vi "Edit Row.vi"(6 "Row Index":i32, 8 "error in (no error)":errorcluster, 9 "New Row Data (or multi rows)":string[][](array[string]), 11 "DataGrid.lvlib:DataTable.lvclass 2":refnum<class "DataTable.lvclass">) -> (0 "error out":errorcluster, 3 "DataGrid.lvlib:DataTable.lvclass 2":refnum<class "DataTable.lvclass">)   [LabVIEW 2016, in "DataGrid.lvlib" / "DataTable.lvclass"]
doc: "Edits a row by simply replacing it with another row (or series of row) to essentially replace and insert at that location in the datatable."
uses:
  <userlib>/LabVIEWdotNetDataGrid/source/DataTable/DataTable.lvclass
  <userlib>/LabVIEWdotNetDataGrid/source/DataTable/DataTable.lvclass/DataTable.ctl
  System.Data
  <userlib>/LabVIEWdotNetDataGrid/source/GridColumn/GridColumn.lvclass/GridColumn.ctl
  <userlib>/LabVIEWdotNetDataGrid/source/GridColumn/Read datatype.vi
  <userlib>/LabVIEWdotNetDataGrid/source/GridColumn/Read Params.vi
  <userlib>/LabVIEWdotNetDataGrid/source/GridColumn/Read Name.vi
  <userlib>/LabVIEWdotNetDataGrid/source/GridColumn/GridColumn.lvclass
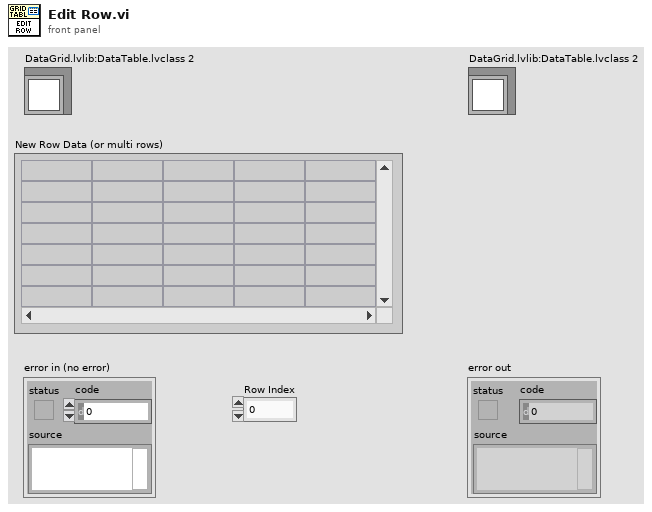
[diagram p1: front panel]
types:
  T1 = typedef "DataGrid.lvlib/GridColumn.lvclass/ColumnType.ctl" = enum16{"string", "image", "check", "numeric", "timestamp", "button", "combo", "link"}
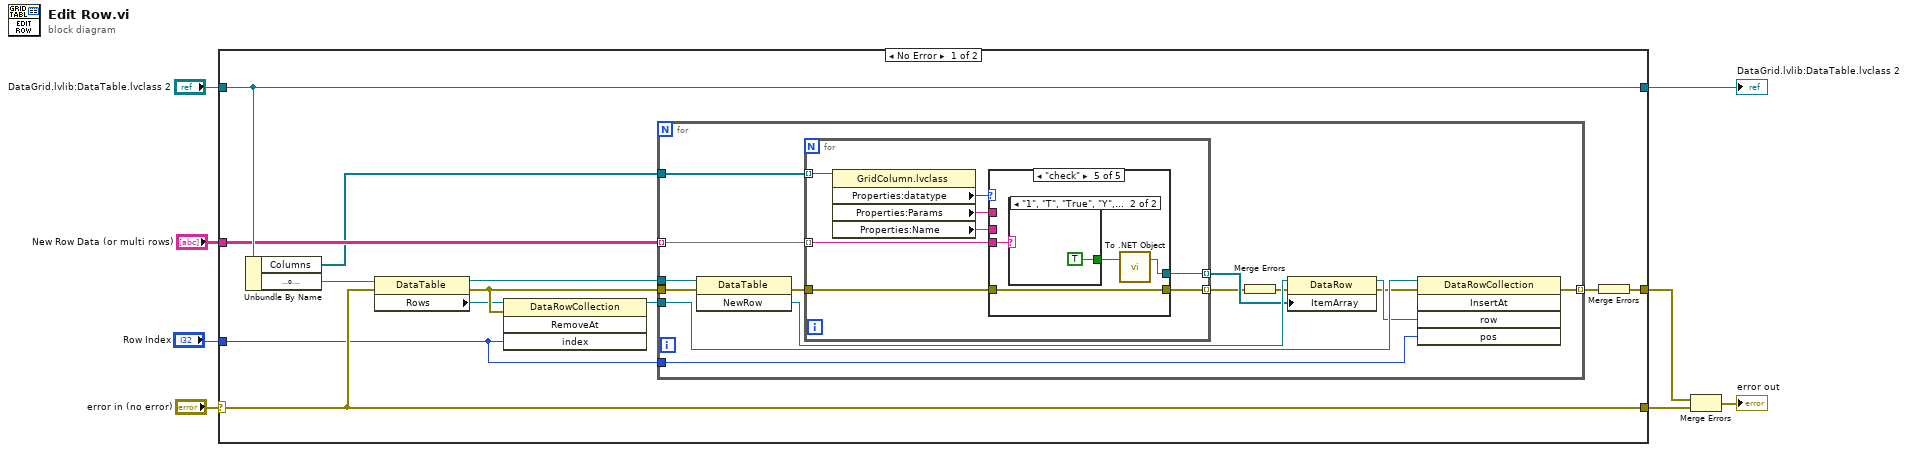
[diagram p0: block diagram]
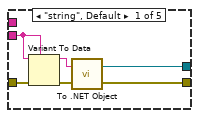
[diagram p2: hidden frame]
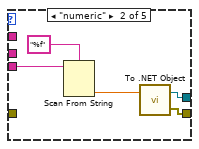
[diagram p3: hidden frame]
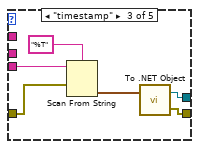
[diagram p4: hidden frame]
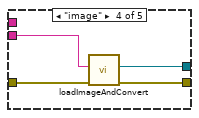
[diagram p5: hidden frame]
diagram:
  n1 = case shown="No Error" "error in (no error)" {
    selector: "error in (no error)" -> [w17 w69]
    tunnel: [w17 w69] -> w7
    tunnel: [w18 w68] -> w5
    tunnel: "DataGrid.lvlib:DataTable.lvclass 2" -> [w18 w68]
    tunnel: "New Row Data (or multi rows)" -> [w16 _]
    tunnel: [w14 _] -> w2
    tunnel: "Row Index" -> [w9 _]
    frame No Error {
      n2 = Unbundle By Name(w18) -> ("Columns"=w13:refnum<class "GridColumn.lvclass">[], "DataTable"=w15:refnum<k24>)
      n3 = property class="DataTable"(reference=w15, error in=w17) -> (reference out=w12:refnum<k24>, error out=w11:errorcluster, "Rows"=w10:refnum<k24>)
      n4 = invoke class="DataRowCollection" method="RemoveAt"(reference=w10, error in=w11, "index"=w9) -> ()  [unwired: 1 in, 4 out]
      n5 = for {
        tunnel: w10 -> [w32]
        tunnel: w12 -> [w33]
        tunnel: [w31] -> w19 mode=indexing
        tunnel: w16 -> [w30] mode=indexing
        tunnel: w11 -> [w22]
        tunnel: w13 -> [w21]
        tunnel: w9 -> [w20]
        n6 = invoke class="DataTable" method="NewRow"(reference=w33, error in=w22) -> (error out=w29:errorcluster, "NewRow"=w28:refnum<k24>)  [unwired: 1 in, 1 out]
        n7 = for {
          tunnel: w30 -> [w41] mode=indexing
          tunnel: [w40] -> w26 mode=indexing
          tunnel: w29 -> [w39]
          tunnel: [w38] -> w25 mode=indexing
          tunnel: w21 -> [w37] mode=indexing
          n8 = property class="GridColumn.lvclass"(reference=w37) -> ("Properties:datatype"=w36:T1, "Properties:Params"=w35:string, "Properties:Name"=w34:string)  [unwired: 1 in, 2 out]
          n9 = case shown="\"check\"" w36 {
            tunnel: w41 -> [w43 w50 w56 w62 w64]
            tunnel: [w42 w51 w57 w61 w65] -> w40
            tunnel: w39 -> [w46 _ w54 w60 w66]
            tunnel: [w44 w52 w58 w59 w66] -> w38
            tunnel: w35 -> [_ _ _ _ _]
            tunnel: w34 -> [_ _ _ _ _]
            frame "string", Default {
              n10 = Variant To Data(error in=w46, type=w43, Variant=w43) -> (data=w47:string, error out=w45:errorcluster)
              n11 = call <vilib>:"To .NET Object.vi"("error in (no error)"=w45, "anything"=w47) -> ("error out"=w44:errorcluster, ".NET object"=w42:refnum<k24>)
            }
            frame "numeric" {
              n12 = Scan From String(format string="%f", input string=w50) -> (output 1=w48:dbl)  [unwired: 3 in, 3 out]
              n13 = call <vilib>:"To .NET Object.vi"("anything"=w48) -> ("error out"=w52:errorcluster, ".NET object"=w51:refnum<k24>)  [unwired: 1 in]
            }
            frame "timestamp" {
              n14 = Scan From String(format string="%T", input string=w56, error in=w54) -> (output 1=w53:timestamp)  [unwired: 2 in, 3 out]
              n15 = call <vilib>:"To .NET Object.vi"("anything"=w53) -> ("error out"=w58:errorcluster, ".NET object"=w57:refnum<k24>)  [unwired: 1 in]
            }
            frame "image" {
              n16 = call <userlib>:"loadImageAndConvert.vi"("error in (no error)"=w60, "name or relative path"=w62) -> ("error out"=w59:errorcluster, ".NET object"=w61:refnum<k24>)  [unwired: 8 in]
            }
            frame "check" {
              n17 = case shown="\"1\", \"T\", \"True\", \"Y\", \"Yes\"" w64 {
                tunnel: [_ TRUE] -> w63
                frame Default {
                }
                frame "1", "T", "True", "Y", "Yes" {
                }
              }
              n18 = call <vilib>:"To .NET Object.vi"("anything"=w63) -> (".NET object"=w65:refnum<k24>)  [unwired: 1 in, 1 out]
            }
          }
        }
        n19 = Merge Errors(w25) -> (w24:errorcluster)
        n20 = property class="DataRow"(reference=w28, error in=w24, "ItemArray"=w26) -> (reference out=w27:refnum<k24>, error out=w23:errorcluster)
        n21 = invoke class="DataRowCollection" method="InsertAt"(reference=w32, error in=w23, "row"=w27, "pos"=w20) -> (error out=w31:errorcluster)  [unwired: 1 in, 4 out]
      }
      n22 = Merge Errors(w19) -> (w14:errorcluster)
    }
    frame Error {
    }
  }
  "DataGrid.lvlib:DataTable.lvclass 2" <- w5
  n23 = Merge Errors(w2, w7) -> (→"error out":errorcluster)
